vi "Configure Control PV Range.vi"(0 "VISA resource name":refnum<visa-resource-name>, 1 "Range Lower Limit":i32=-270, 5 "Loop No. String":string="L001", 7 "Decimal Point":i32=1, 9 "Unit String":string, 11 "error in (no error)":errorcluster, 13 "Range Upper Limit":i32=1370) -> (4 "VISA resource name out":refnum<visa-resource-name>, 15 "error out":errorcluster)   [LabVIEW 2020, in "Yokogawa GX Series.lvlib"]
doc: "Set PV range.\n\nCommand: SCtrlRangePV"
uses:
  <instrlib>/Yokogawa GX Series/Yokogawa GX Series.lvlib
panel:
  out "Loop No. String":string
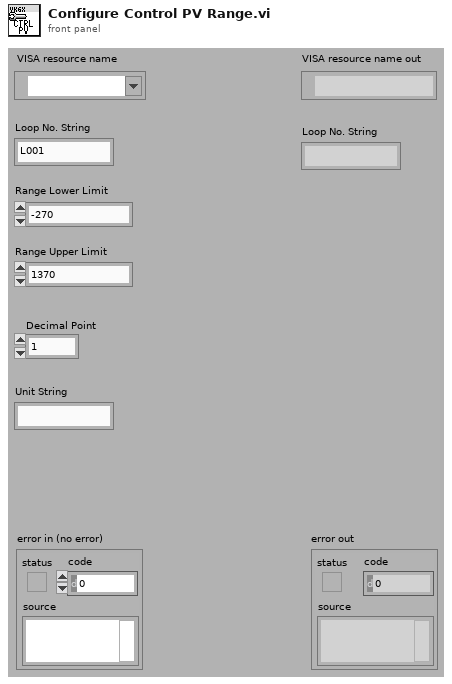
[diagram p1: front panel]
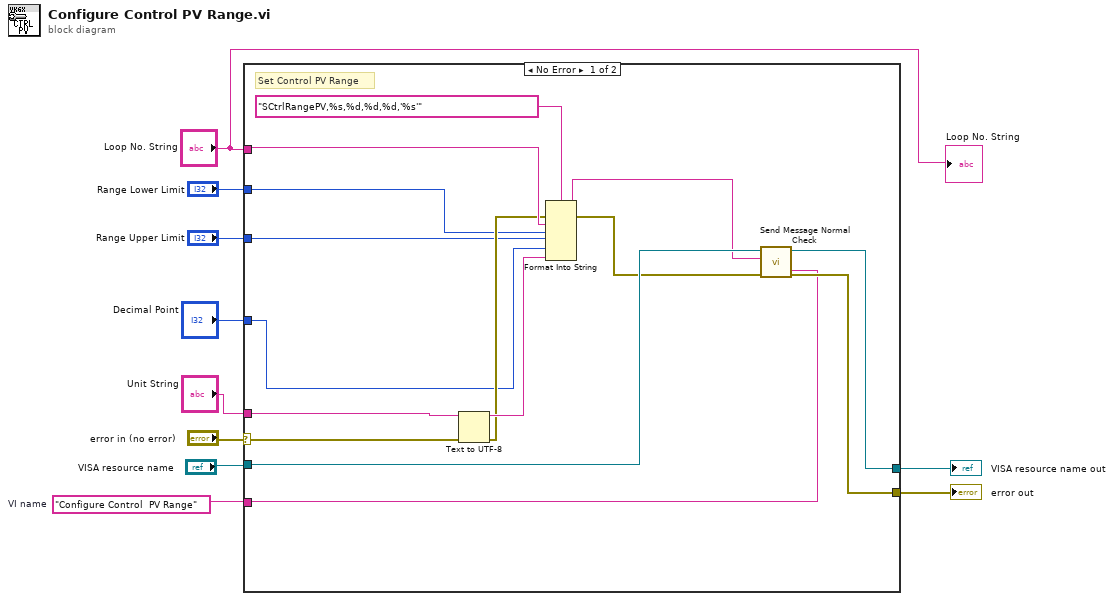
[diagram p0: block diagram]
diagram:
  w6 = "Configure Control  PV Range"  # VI name
  n1 = case shown="No Error" "error in (no error)" {
    selector: "error in (no error)" -> [w15 w26]
    tunnel: [w25 w27] -> w10
    tunnel: [w24 w26] -> w9
    tunnel: "VISA resource name" -> [w23 w27]
    tunnel: w6 -> [w21 _]
    tunnel: "Loop No. String" -> [w20 _]
    tunnel: "Range Lower Limit" -> [w12 _]
    tunnel: "Range Upper Limit" -> [w11 _]
    tunnel: "Decimal Point" -> [w13 _]
    tunnel: "Unit String" -> [w17 _]
    frame No Error {
      # "Set Control PV Range"
      n2 = Text to UTF-8(8:w15, 11:w17) -> (0:w14:errorcluster, 3:w16:string)  [unwired: 1 in]
      n3 = Format Into String(format string="SCtrlRangePV,%s,%d,%d,%d,'%s'", error in=w14, w20, w12, w11, w13, w16) -> (resulting string=w18:string, error out=w19:errorcluster)  [unwired: 1 in]
      n4 = call <instrlib>:"Send Message Normal Check.vi"("Source (\"\")"=w21, "error in (no error)"=w19, "Send Message (\"\")"=w18, "VISA resource name"=w23) -> ("error out"=w24:errorcluster, "VISA resource name out"=w25:refnum<visa-resource-name>)  [unwired: 2 in, 4 out]
    }
    frame Error {
    }
  }
  "error out" <- w9
  "VISA resource name out" <- w10
  "Loop No. String" <- "Loop No. String"
